vi "Arena Settings from ini.vi"(7 "Section":string, 8 "error in (no error)":errorcluster) -> (0 "error out":errorcluster, 3 "Arena filepath":path, 5 "All Tags Exists?":bool)   [LabVIEW 2013]
doc: "Loads the arena config file root path from the ini."
uses:
  Arena Enum Keys.ctl
  Common/File IO/INI/Read write mode.ctl
  HHMI - Filepaths global.vi
  Common/File IO/INI/INI Read write path.vi
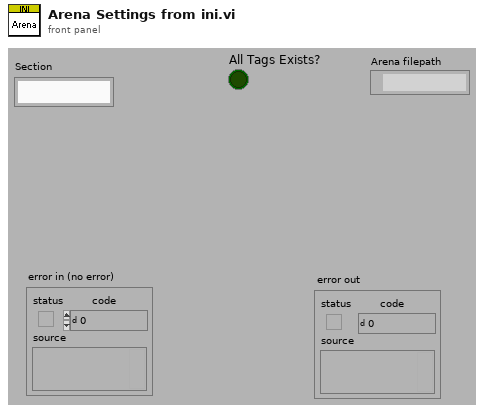
[diagram p1: front panel]
types:
  T1 = typedef "Arena Enum Keys.ctl" = enum16{"Path"}
  T2 = typedef "Read write mode.ctl" = enum16{"Read", "Write"}
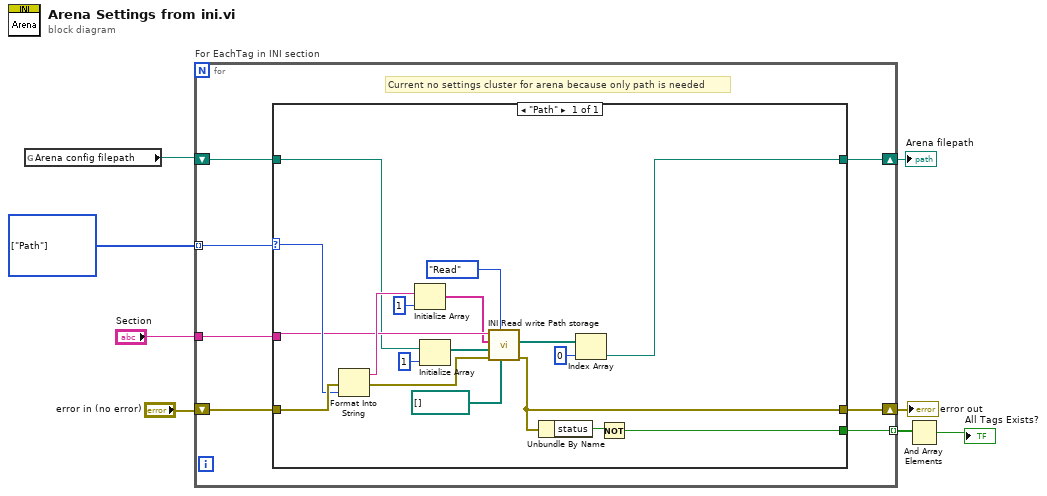
[diagram p0: block diagram]
diagram:
  w8 = T1[] [enum."Path"] items=["Path"]
  n1 = global read "HHMI - Filepaths global.vi" "Arena config filepath"() -> (w2:path)
  n2 = for "For EachTag in INI section" {
    tunnel: "Section" -> [w15]
    tunnel: w8 -> [w14] mode=indexing
    shift-right: [w9] -> w6
    shift-left: "error in (no error)" -> [w12]
    shift-right: [w10] -> w1
    shift-left: w2 -> [w13]
    tunnel: [w11] -> w4 mode=indexing
    # "Current no settings cluster for arena because only path is needed"
    n3 = case shown="\"Path\"" w14 {
      selector: w14 -> [w32]
      tunnel: w15 -> [w25]
      tunnel: w13 -> [w23]
      tunnel: w12 -> [w33]
      tunnel: [w27] -> w11
      tunnel: [w18] -> w10
      tunnel: [w17] -> w9
      frame "Path" {
        n4 = Format Into String(error in=w33, w32) -> (resulting string=w30:string, error out=w21:errorcluster)  [unwired: 2 in]
        n5 = Initialize Array(w30, 1 ("dimension size")) -> (w24:string[])
        n6 = Initialize Array(w23, 1 ("dimension size")) -> (w22:path[])
        n7 = call "INI Read write Path storage.vi"("Values to write"=path[] [], "Read/Write mode"=Read_write_mode."Read", "error in"=w21, "Defaults"=w22, "keys"=w24, "section"=w25) -> ("error out"=w17:errorcluster, "Values"=w19:path[])  [unwired: 4 in]
        n8 = Unbundle By Name(w17) -> ("status"=w16:bool)
        n9 = Index Array(array=w19, index=0) -> (element=w18:path)
        n10 = Not(x=w16) -> (.not. x?=w27:bool)
      }
    }
  }
  "error out" <- w6
  "Arena filepath" <- w1
  n11 = And Array Elements(Boolean array=w4) -> (logical AND=→"All Tags Exists?":bool)
